vi "test Reading an Already Read Result Gets The Same Result.vi"(8 "error in (no error)":errorcluster, 11 "TestCase in":refnum<class "Result Tests.lvclass">) -> (0 "error out":errorcluster, 3 "TestCase out":refnum<class "Result Tests.lvclass">)   [LabVIEW 2017, in "Result Tests.lvclass"]
uses:
  Result Tests.lvclass
  <vilib>/addons/_JKI Toolkits/VI Tester/TestCase.llb/TestCase.lvclass
  Futures/Result/Result.lvclass
  C:/Program Files (x86)/National Instruments/LabVIEW 2017/vi.lib/addons/_JKI Toolkits/VI Tester/TestCase.llb/TestCase.lvclass
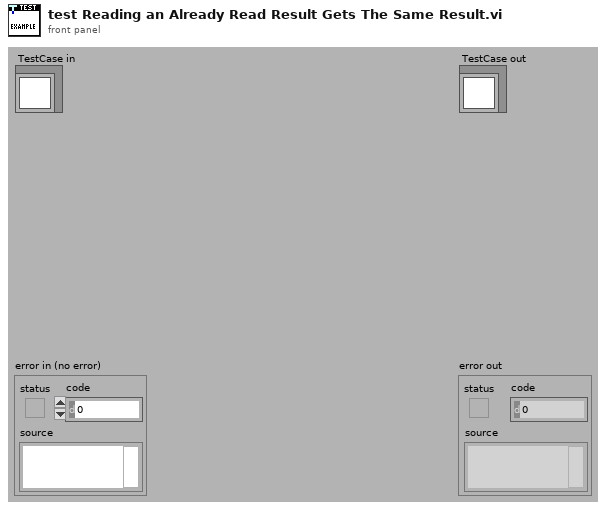
[diagram p1: front panel]
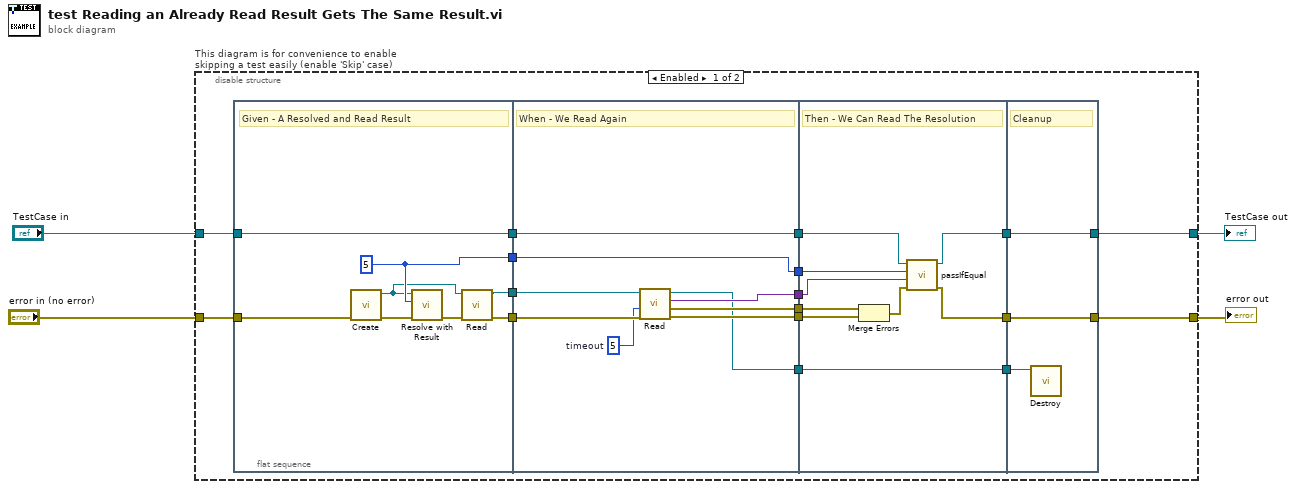
[diagram p0: block diagram]
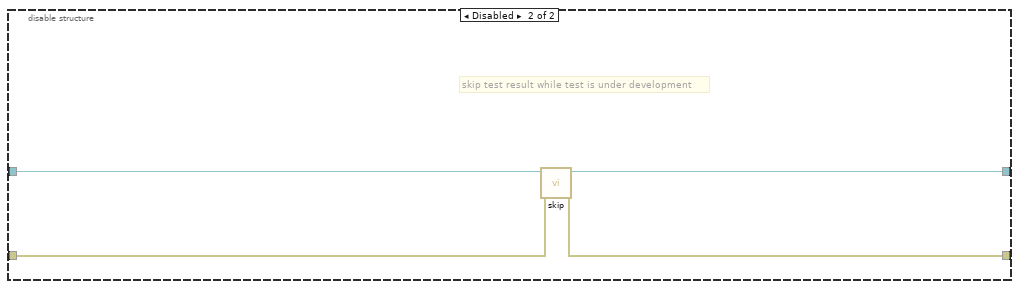
[diagram p2: hidden frame]
diagram:
  n1 = disable-structure "This diagram is for convenience to enable skipping a test easily (enable 'Skip' case)" shown="Enabled" {
    disable-tunnel: "TestCase in" -> [w17 w54]
    disable-tunnel: [w15 w52] -> w1
    disable-tunnel: [w14 w53] -> w3
    disable-tunnel: "error in (no error)" -> [w16 w51]
    frame Enabled {
      n2 = flat-sequence {
        tunnel: w16 -> [w28]
        tunnel: w17 -> [w29]
        tunnel: [w29] -> w21
        tunnel: [w26] -> w12
        tunnel: [w24] -> w8
        tunnel: [w22] -> w7
        tunnel: [w38] -> w20
        tunnel: w21 -> [w38]
        tunnel: [w37] -> w13
        tunnel: w12 -> [w37]
        tunnel: [w36] -> w11
        tunnel: [w35] -> w10
        tunnel: [w34] -> w9
        tunnel: w8 -> [w33]
        tunnel: w7 -> [w32]
        tunnel: [w31] -> w6
        tunnel: [w46] -> w19
        tunnel: [w45] -> w18
        tunnel: w20 -> [w47]
        tunnel: w13 -> [w43]
        tunnel: w11 -> [w42]
        tunnel: w10 -> [w41]
        tunnel: w9 -> [w40]
        tunnel: w6 -> [w39]
        tunnel: [w39] -> w5
        tunnel: [w49] -> w14
        tunnel: [w50] -> w15
        tunnel: w19 -> [w50]
        tunnel: w18 -> [w49]
        tunnel: w5 -> [w48]
        frame #0 {
          w26 = 5
          # "Given - A Resolved and Read Result"
          n3 = call "Create.vi"("error in (no error)"=w28) -> ("error out"=w27:errorcluster, "Result out"=w23:refnum<class "Result.lvclass">)  [unwired: 9 in]
          n4 = call "Resolve with Result.vi"("error in (no error)"=w27, "Result"=w26, "Result in"=w23) -> ("error out"=w25:errorcluster)  [unwired: 8 in]
          n5 = call "Read.vi"("error in (no error)"=w25, "Result in"=w23) -> ("error out"=w24:errorcluster, "Result Out"=w22:refnum<class "Result.lvclass">)  [unwired: 5 in, 3 out]
        }
        frame #1 {
          w30 = 5  # timeout
          # "When - We Read Again"
          n6 = call "Read.vi"("error in (no error)"=w33, "timeout in ms (-1)"=w30, "Result in"=w32) -> ("error out"=w36:errorcluster, "result error"=w35:errorcluster, "Result value"=w34:variant, "Result Out"=w31:refnum<class "Result.lvclass">)  [unwired: 4 in, 1 out]
        }
        frame #2 {
          # "Then - We Can Read The Resolution"
          n7 = Merge Errors(w41, w42) -> (w44:errorcluster)
          n8 = call-dynamic "passIfEqual.vi"("error in (no error)"=w44, "y"=w40, "x"=w43, "TestCase in"=w47) -> ("error out"=w45:errorcluster, "TestCase out"=w46:refnum<class "Result Tests.lvclass">)  [unwired: 6 in]
        }
        frame #3 {
          # "Cleanup"
          n9 = call "Destroy.vi"("Result in"=w48) -> ()  [unwired: 10 in, 1 out]
        }
      }
    }
    frame Disabled {
      # "skip test result while test is under development"
      n10 = call <vilib>:"skip.vi"("error in (no error)"=w51, "TestCase in"=w54) -> ("error out"=w53:errorcluster, "TestCase out"=w52:refnum<class "Result Tests.lvclass">)  [unwired: 8 in]
    }
  }
  "error out" <- w3
  "TestCase out" <- w1
